vi "원격제어 명령.vi"() -> ()   [LabVIEW 2014]
panel:
  in  "확인 버튼":bool
  in  "address":string="127.0.0.1"
  out "명령코드":i16[](array[numeric])
  in  "불리언":bool
  out "참 거짓":string
  out "문자열":string
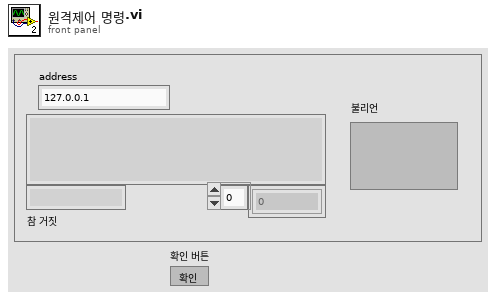
[diagram p1: front panel]
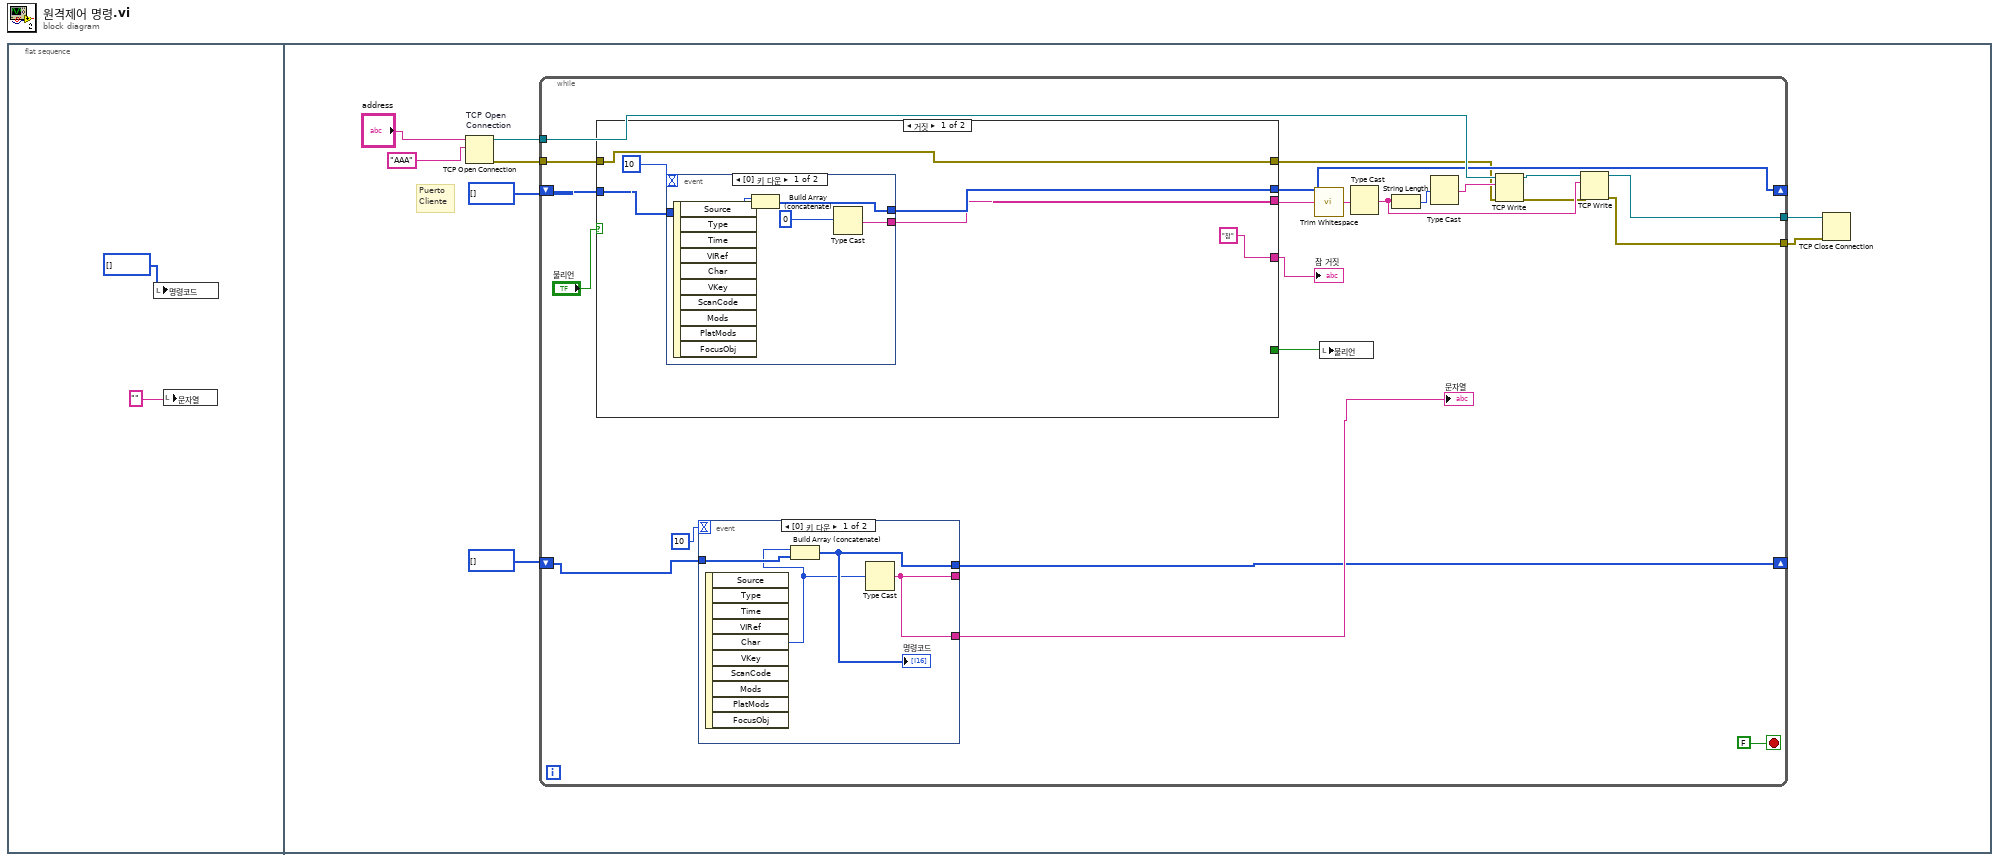
[diagram p0: block diagram]
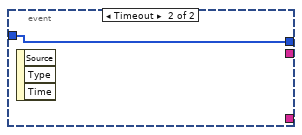
[diagram p2: hidden frame]
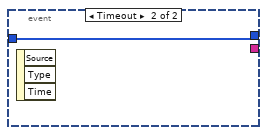
[diagram p3: hidden frame]
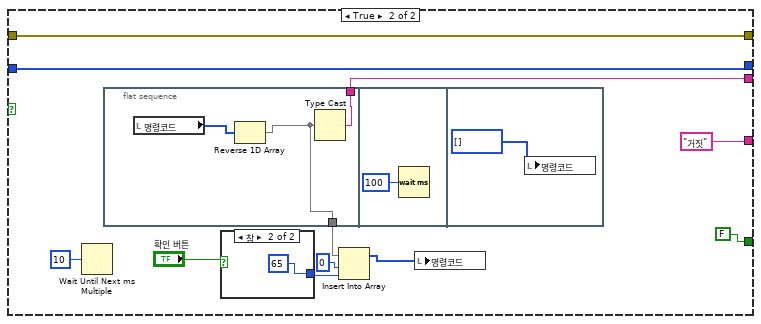
[diagram p4: hidden frame]
diagram:
  n1 = flat-sequence {
    frame #0 {
      n2 = local write "명령코드"(i16[] []) -> ()
      n3 = local write "문자열"("") -> ()
    }
    frame #1 {
      # "Puerto\nCliente"
      n4 = TCP Open Connection "TCP Open \nConnection"(address="address", remote port or service name="AAA") -> (connection ID=w10:refnum<k5>, error out=w6:errorcluster)  [unwired: 3 in]
      n5 = while {
        tunnel: w10 -> [w30]
        tunnel: [w32] -> w9
        shift-right: [w19] -> _
        shift-left: i16[] [] -> [w31]
        shift-right: [w20] -> _
        shift-left: i16[] [] -> [w21]
        tunnel: w6 -> [w18]
        tunnel: [w15] -> w5
        stop <- FALSE stop-if-true
        n6 = case shown="거짓" "불리언" {
          tunnel: w31 -> [w43 w60]
          tunnel: [w42 w60] -> w19
          tunnel: [_ FALSE ("불리언")] -> w24
          tunnel: [w40 w55] -> w13
          tunnel: w18 -> [w39 w57]
          tunnel: [w39 w57] -> w17
          tunnel: ["참" "거짓"] -> w12
          frame False {
            n7 = event shown="[0] 키 다운" {
              selector: _ -> [_ _]
              dyn-events: _ -> [_ _]
              timeout: 10 -> [_ _]
              tunnel: [w47 w49] -> w42
              tunnel: w43 -> [w48 w49]
              tunnel: [w45 _] -> w40
              event Key Down {
                n8 = event-data() -> ("Char"=w46:i16)  [unwired: 1 in, 9 out]
                n9 = Build Array (concatenate)(w46, w48) -> (w47:i16[])
                n10 = Type Cast(x=0) -> (*(type *) &x=w45:string)  [unwired: 1 in]
              }
              event Timeout {
                n11 = event-data() -> ()  [unwired: 1 in, 3 out]
              }
            }
          }
          frame True {
            n12 = Wait Until Next ms Multiple(millisecond multiple=u32 10) -> ()  [unwired: 1 out]
            n13 = flat-sequence {
              tunnel: [w63] -> w55
              tunnel: [w62] -> w53
              frame #0 {
                n14 = local read "명령코드"() -> (w64:i16[])
                n15 = Reverse 1D Array(array=w64) -> (reversed array=w62:i16[])
                n16 = Type Cast(x=w62) -> (*(type *) &x=w63:string)  [unwired: 1 in]
              }
              frame #1 {
                n17 = Wait (ms)(milliseconds to wait=u32 100 ("대기 시간(ms)")) -> ()  [unwired: 1 out]
              }
              frame #2 {
                n18 = local write "명령코드"(i16[] []) -> ()
              }
            }
            n19 = case shown="참" "확인 버튼" {
              tunnel: [_ i16 65] -> w52
              frame False {
              }
              frame True {
              }
            }
            n20 = Insert Into Array(array=w53, index=0 ("인덱스"), new element=w52) -> (w50:i16[])
            n21 = local write "명령코드"(w50) -> ()
          }
        }
        "참 거짓" <- w12
        n22 = event shown="[0] 키 다운" {
          selector: _ -> [_ _]
          dyn-events: _ -> [_ _]
          timeout: 10 -> [_ _]
          tunnel: [w34 w37] -> w20
          tunnel: [w36 _] -> w22
          tunnel: [w36 _] -> _
          tunnel: w21 -> [w35 w37]
          event Key Down {
            n23 = event-data() -> ("Char"=w33:i16)  [unwired: 1 in, 9 out]
            n24 = Build Array (concatenate)(w33, w35) -> (w34:i16[])
            "명령코드" <- w34
            n25 = Type Cast(x=w33) -> (*(type *) &x=w36:string)  [unwired: 1 in]
          }
          event Timeout {
            n26 = event-data() -> ()  [unwired: 1 in, 3 out]
          }
        }
        "문자열" <- w22
        n27 = call <vilib>:"Trim Whitespace.vi"("string"=w13) -> ("trimmed string"=w14:string)  [unwired: 1 in]
        n28 = local write "불리언"(w24) -> ()
        n29 = Type Cast(x=w14) -> (*(type *) &x=w26:string)  [unwired: 1 in]
        n30 = String Length(string=w26) -> (length=w27:i32)
        n31 = Type Cast(x=w27) -> (*(type *) &x=w28:string)  [unwired: 1 in]
        n32 = TCP Write(connection ID=w30, data in=w28, error in (no error)=w17) -> (connection ID out=w29:refnum<k5>, error out=w16:errorcluster)  [unwired: 1 in, 1 out]
        n33 = TCP Write(connection ID=w29, data in=w26, error in (no error)=w16) -> (connection ID out=w32:refnum<k5>, error out=w15:errorcluster)  [unwired: 1 in, 1 out]
      }
      n34 = TCP Close Connection(connection ID=w9, error in (no error)=w5) -> ()  [unwired: 1 in, 2 out]
    }
  }
